vi "provide_note_book_info.vi"(8 "error in (no error)":errorcluster, 10 "notebook string in":string, 11 "GenericPlugin in":refnum<class "ImagingModeMG090624Camera.lvclass">) -> (0 "error out":errorcluster, 2 "notebook string out":string, 3 "GenericPlugin out":refnum<class "ImagingModeMG090624Camera.lvclass">)   [LabVIEW 2010, in "ImagingModeMG090624Camera.lvclass"]
uses:
  ImagingModeMG090624Camera.lvclass
  ImagingModeDL091001Scaffold/ImagingModeDL091001Scaffold/ImagingModeDL091001Scaffold.lvclass
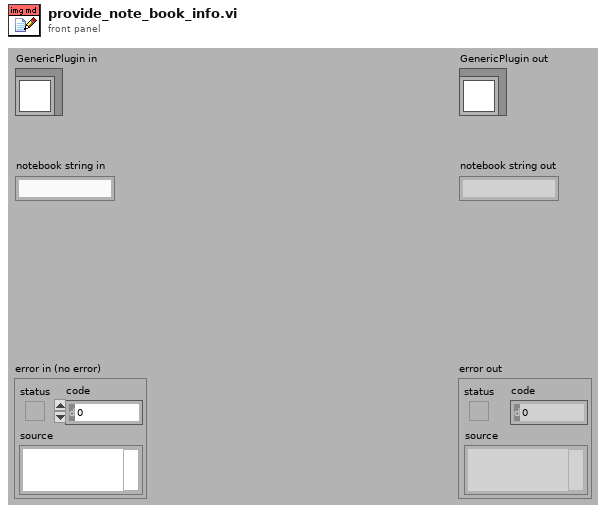
[diagram p1: front panel]
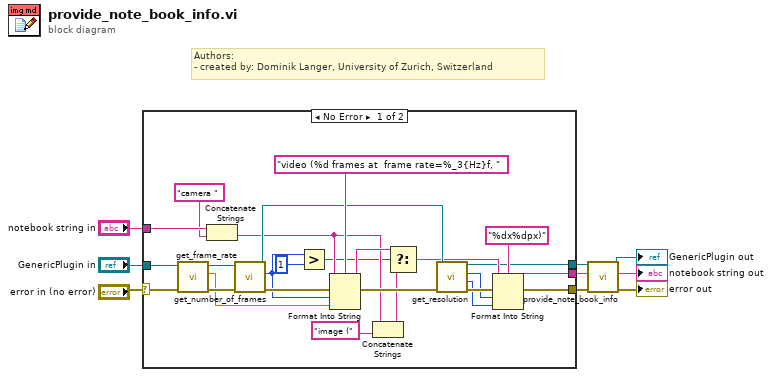
[diagram p0: block diagram]
diagram:
  # "Authors: \n- created by: Dominik Langer, University of Zurich, Switzerland"
  n1 = case shown="No Error" "error in (no error)" {
    selector: "error in (no error)" -> [w19 w37]
    tunnel: [w27 w37] -> w5
    tunnel: "notebook string in" -> [w15 w36]
    tunnel: "GenericPlugin in" -> [w21 w38]
    tunnel: [w22 w38] -> w2
    tunnel: [w16 w36] -> w1
    frame No Error {
      n2 = call-dynamic "get_frame_rate.vi"("error in (no error)"=w19, "ScanModeMG090624Camera in"=w21) -> ("error out"=w18:errorcluster, "frame rate"=w17:dbl[unit], "ScanModeMG090624Camera out"=w20:refnum<class "ImagingModeMG090624Camera.lvclass">)  [unwired: 7 in]
      n3 = Concatenate Strings(w15, "camera " ("string")) -> (w13:string)
      n4 = call-dynamic "get_number_of_frames.vi"("error in (no error)"=w18, "ScanModeMG090624Camera in"=w20) -> ("error out"=w35:errorcluster, "number of frames"=w33:i32, "ScanModeMG090624Camera out"=w29:refnum<class "ImagingModeMG090624Camera.lvclass">)  [unwired: 7 in]
      n5 = Greater?(x=w33, y=1) -> (0:w11:bool)
      n6 = Format Into String(format string="video (%d frames at  frame rate=%_3{Hz}f, ", initial string=w13, error in=w35, w33, w17) -> (resulting string=w31:string, error out=w30:errorcluster)
      n7 = Concatenate Strings(w13, "image (") -> (w10:string)
      n8 = Select(t=w31, s=w11, f=w10) -> (s? t:f=w24:string)
      n9 = call-dynamic "get_resolution.vi"("error in (no error)"=w30, "ScanModeMG090624Camera in"=w29) -> ("error out"=w28:errorcluster, "y"=w25:i32, "x"=w26:i32, "ScanModeMG090624Camera out"=w22:refnum<class "ImagingModeMG090624Camera.lvclass">)  [unwired: 6 in]
      n10 = Format Into String(format string="%dx%dpx)", initial string=w24, error in=w28, w26, w25) -> (resulting string=w16:string, error out=w27:errorcluster)
    }
    frame Error {
    }
  }
  n11 = call-parent "provide_note_book_info.vi"("error in (no error)"=w5, "notebook string in"=w1, "GenericPlugin in"=w2) -> ("error out"=→"error out":errorcluster, "notebook string out"=→"notebook string out":string, "GenericPlugin out"=→"GenericPlugin out":refnum<class "ImagingModeMG090624Camera.lvclass">)  [unwired: 6 in]
